vi "getFeedback.vi"(0 "Interface in":T2, 5 "timeout (5000 ms)":i32=5000, 11 "error in":errorcluster) -> (4 "Interface out":T2, 6 "feedback":T1, 15 "error out":errorcluster)   [LabVIEW 2017, in "AFE_interface.lvlib"]
uses:
  AFE_interface.lvlib
  InterfaceRef.ctl
  <instrlib>/_niInstr/Instruction Framework/v1/Host/Instruction Target/niInstr Instruction Target v1 Host.lvclass
  <instrlib>/_niInstr/Instruction Framework/v1/Host/Instruction Framework Context/niInstr Instruction Framework Context v1 Host.lvclass
  Feedback.ctl
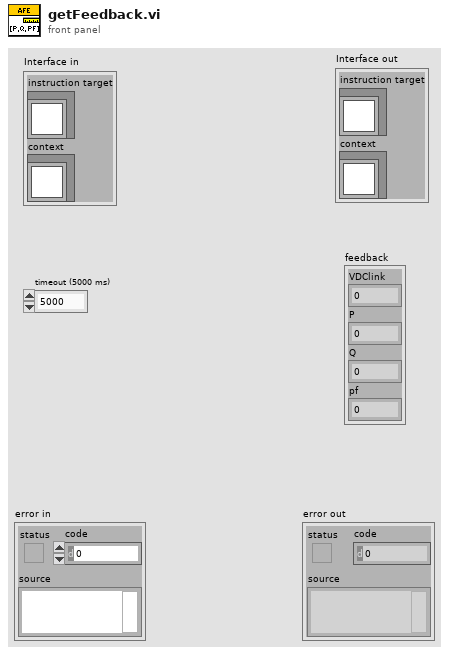
[diagram p1: front panel]
types:
  T1 = typedef "AFE_interface.lvlib/Feedback.ctl" = cluster{"VDClink":dbl, "P":dbl, "Q":dbl, "pf":dbl}
  T2 = typedef "AFE_interface.lvlib/InterfaceRef.ctl" = cluster{"instruction target":refnum<class "niInstr Instruction Target v1 Host.lvclass">, "context":refnum<class "niInstr Instruction Framework Context v1 Host.lvclass">}
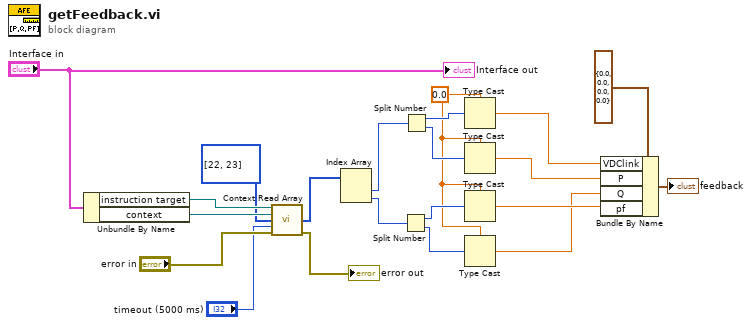
[diagram p0: block diagram]
diagram:
  w7 = sgl 0.0
  n1 = Unbundle By Name("Interface in") -> ("instruction target"=w21:refnum<class "niInstr Instruction Target v1 Host.lvclass">, "context"=w20:refnum<class "niInstr Instruction Framework Context v1 Host.lvclass">)
  n2 = call <instrlib>:"Context Read Array.vi"("instruction target in"=w21, "context in"=w20, "addresses"=u64[] [22, 23], "timeout (5000 ms)"="timeout (5000 ms)", "error in"="error in") -> ("data"=w14:u64[], "error out"=→"error out":errorcluster)  [unwired: 7 in, 2 out]
  n3 = Index Array(array=w14) -> (element #1=w13:u64, element #2=w12:u64)  [unwired: 2 in]
  n4 = Split Number(x=w12) -> (hi(x)=w9:u32, lo(x)=w8:u32)
  n5 = Split Number(x=w13) -> (hi(x)=w11:u32, lo(x)=w10:u32)
  n6 = Type Cast(type=w7, x=w11) -> (*(type *) &x=w5:sgl)
  n7 = Type Cast(type=w7, x=w10) -> (*(type *) &x=w4:sgl)
  n8 = Type Cast(type=w7, x=w9) -> (*(type *) &x=w3:sgl)
  n9 = Type Cast(type=w7, x=w8) -> (*(type *) &x=w2:sgl)
  n10 = Bundle By Name(cluster=T1 {"VDClink"=0.0, "P"=0.0, "Q"=0.0, "pf"=0.0} ("Feedback"), "VDClink"=w5, "P"=w4, "Q"=w2, "pf"=w3) -> (→"feedback":T1)
  "Interface out" <- "Interface in"
